vi "Finish.vi"(4 "error in":errorcluster) -> ()   [LabVIEW 2013]
doc: "This VI is called just before exiting. It is expected to close I/O refnum, save collected data, etc."
uses:
  <vilib>/Rock Robotics/WPI/Solenoid/WPI_SolenoidValue.ctl
  <vilib>/Rock Robotics/WPI/RobotDrive/WPI_RobotDriveGetSetRefNum.vi
  <vilib>/Rock Robotics/WPI/Joystick/WPI_JoystickGetSetRefNum.vi
  <vilib>/Rock Robotics/WPI/Solenoid/WPI_SolenoidSetEnum.vi
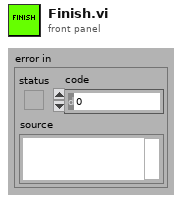
[diagram p1: front panel]
types:
  T1 = typedef "WPI_DigitalInputDevRef.ctl" = cluster{"DevStatus":errorcluster, "DIO Channel":T2, "Digital Module":T3}
  T2 = typedef "FPGA_DIOChannel.ctl" = enum8{"DIO 1", "DIO 2", "DIO 3", "DIO 4", "DIO 5", "DIO 6", "DIO 7", "DIO 8", "DIO 9", "DIO 10", "DIO 11", "DIO 12", "DIO 13", "DIO 14", "Invalid"}
  T3 = typedef "FPGA_TypedefDigitalModule.ctl" = enum16{"Digital Module 1", "Digital Module 2"}
  T4 = typedef "WPI_JoystickDevRef.ctl" = cluster{"Device":T5}
  T5 = typedef "WPI_JoystickDeviceEnum.ctl" = enum16{"USB 1", "USB 2", "USB 3", "USB 4", "Kinect 1", "Kinect 2"}
  T6 = typedef "WPI_CameraDevRef.ctl" = cluster{"Camera Address":string, "CameraStatus":errorcluster, "Acquire Image Notifier":refnum<notifier>}
  T7 = typedef "WPI_RobotDriveDevRef.ctl" = cluster{"DevStatus":errorcluster, "Motors[]":T8[], "Square Inputs":bool, "Max Output":dbl, "Isochronous":bool}
  T8 = typedef "WPI_MotorControlDeviceRef.ctl" = cluster{"DeviceStatus":errorcluster, "Type":enum16{"PWM", "CAN"}, "PWM":cluster{"Digital Module":T3, "PWM Channel":T9, "DeadBand":T10}, "CAN":cluster{"Device Number":u8, "Control Mode":T11, "Semaphore":T12, "Max Vout":dbl}, "Invert":bool, "TransformRef":T13, "InvTransformRef":T13}
  T9 = typedef "FPGA_DIOPWMChannel.ctl" = enum8{"PWM 1", "PWM 2", "PWM 3", "PWM 4", "PWM 5", "PWM 6", "PWM 7", "PWM 8", "PWM 9", "PWM 10", "Invalid"}
  T10 = typedef "WPI_PWMDeadband.ctl" = cluster{"Name":string, "maxPositivePwm":i32, "minPositivePwm":i32, "centerPwm":i32, "maxNegativePwm":i32, "minNegativePwm":i32, "angularRange":u16}
  T11 = typedef "WPI_CANJaguar_ControlMode.ctl" = enum8{"Percent VBus", "Current", "Speed", "Position", "Voltage"}
  T12 = typedef "Semaphore RefNum" = refnum<k1>
  T13 = typedef "WPI_PWMTransform_ConPane.ctl" = refnum<vi>
  T14 = typedef "WPI_EncoderDevRef.ctl" = cluster{"DevStatus":errorcluster, "EncoderIndex":T15, "CounterIndex":T16, "DistancePerCount":dbl, "Decoding Type":T17}
  T15 = typedef "FPGA_EncoderIdx.ctl" = enum8{"Enc 0", "Enc 1", "Enc 2", "Enc 3", "Invalid"}
  T16 = typedef "FPGA_CounterCtrSystemIndex.ctl" = enum8{"Ctr 0", "Ctr 1", "Ctr 2", "Ctr 3", "Ctr 4", "Ctr 5", "Ctr 6", "Ctr 7", "Invalid"}
  T17 = typedef "WPI_EncoderType.ctl" = enum16{"1x", "2x", "4x"}
  T18 = typedef "WPI_SolenoidDevRef.ctl" = cluster{"DevStatus":errorcluster, "Solenoid Module":T19, "Forward Solenoid Channel":T20, "Reverse Solenoid Channel":T20}
  T19 = typedef "FPGA_TypedefSolenoidModule.ctl" = enum16{"Solenoid Module 1", "Solenoid Module 2"}
  T20 = typedef "WPI_SolenoidChannel.ctl" = enum8{"Solenoid 1", "Solenoid 2", "Solenoid 3", "Solenoid 4", "Solenoid 5", "Solenoid 6", "Solenoid 7", "Solenoid 8", "Invalid"}
  T21 = typedef "WPI_SolenoidValue.ctl" = enum16{"Off", "On", "Forward", "Reverse"}
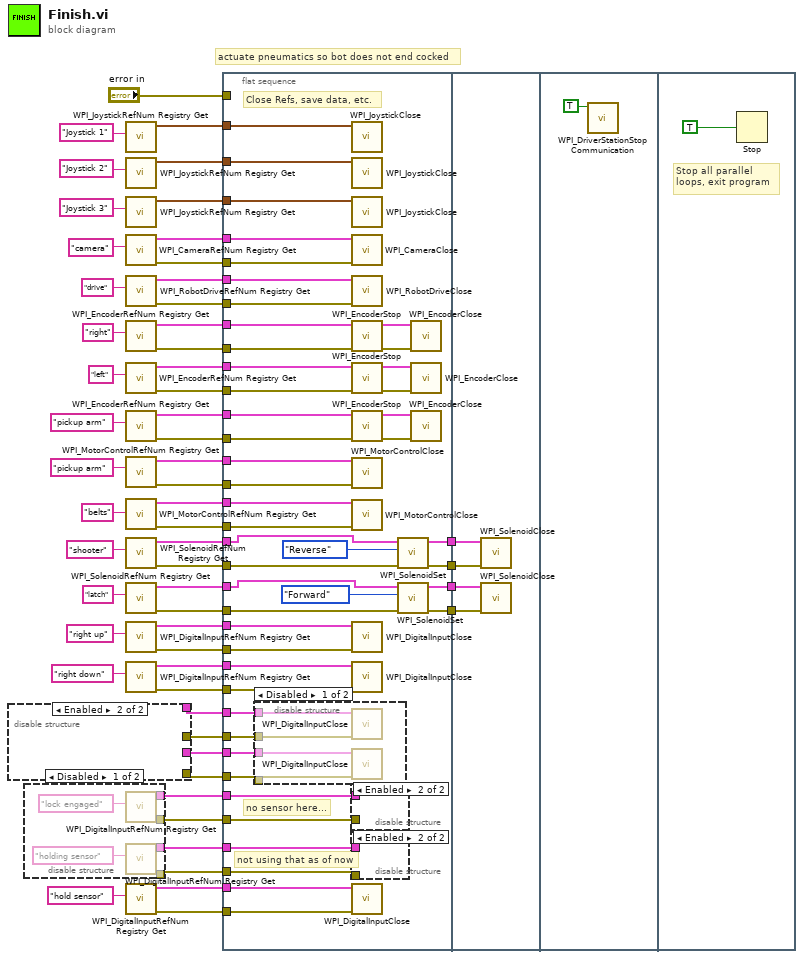
[diagram p0: block diagram]
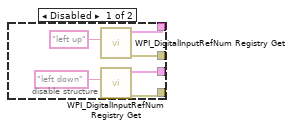
[diagram p2: hidden frame]
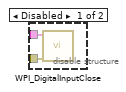
[diagram p5: hidden frame]
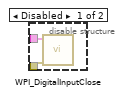
[diagram p6: hidden frame]
diagram:
  # "actuate pneumatics so bot does not end cocked"
  n1 = disable-structure shown="Enabled" {
    disable-tunnel: [w59 _] -> w15
    disable-tunnel: [w58 _] -> w14
    disable-tunnel: [w57 _] -> w13
    disable-tunnel: [w56 _] -> w12
    frame Disabled {
      n2 = call <vilib>:"WPI_DigitalInputRefNum Registry Get.vi"("refnum name"="left up") -> ("error out"=w58:errorcluster, "DigitalInputDevRef"=w59:T1)  [unwired: 9 in]
      n3 = call <vilib>:"WPI_DigitalInputRefNum Registry Get.vi"("refnum name"="left down") -> ("error out"=w56:errorcluster, "DigitalInputDevRef"=w57:T1)  [unwired: 9 in]
    }
    frame Enabled {
    }
  }
  n4 = disable-structure shown="Disabled" {
    disable-tunnel: [w67 _] -> w9
    disable-tunnel: [w66 _] -> w8
    disable-tunnel: [w64 _] -> w6
    disable-tunnel: [w63 _] -> w5
    frame Disabled {
      n5 = call <vilib>:"WPI_DigitalInputRefNum Registry Get.vi"("refnum name"="lock engaged") -> ("error out"=w64:errorcluster, "DigitalInputDevRef"=w63:T1)  [unwired: 9 in]
      n6 = call <vilib>:"WPI_DigitalInputRefNum Registry Get.vi"("refnum name"="holding sensor") -> ("error out"=w67:errorcluster, "DigitalInputDevRef"=w66:T1)  [unwired: 9 in]
    }
    frame Enabled {
    }
  }
  n7 = call <vilib>:"WPI_JoystickRefNum Registry Get.vi"("refnum name"="Joystick 1") -> ("JoystickDevRef"=w54:T4)  [unwired: 1 in, 9 out]
  n8 = call <vilib>:"WPI_JoystickRefNum Registry Get.vi"("refnum name"="Joystick 2") -> ("JoystickDevRef"=w51:T4)  [unwired: 1 in, 9 out]
  n9 = call <vilib>:"WPI_JoystickRefNum Registry Get.vi"("refnum name"="Joystick 3") -> ("JoystickDevRef"=w48:T4)  [unwired: 1 in, 9 out]
  n10 = call <vilib>:"WPI_CameraRefNum Registry Get.vi"("refnum name"="camera") -> ("error out"=w41:errorcluster, "CameraDevRef"=w53:T6)  [unwired: 1 in, 8 out]
  n11 = call <vilib>:"WPI_RobotDriveRefNum Registry Get.vi"("refnum name"="drive") -> ("error out"=w40:errorcluster, "RobotDriveDevRef"=w46:T7)  [unwired: 9 in]
  n12 = call <vilib>:"WPI_EncoderRefNum Registry Get.vi"("refnum name"="right") -> ("error out"=w39:errorcluster, "EncoderDevRef"=w43:T14)  [unwired: 9 in]
  n13 = call <vilib>:"WPI_EncoderRefNum Registry Get.vi"("refnum name"="left") -> ("error out"=w38:errorcluster, "EncoderDevRef"=w42:T14)  [unwired: 9 in]
  n14 = call <vilib>:"WPI_EncoderRefNum Registry Get.vi"("refnum name"="pickup arm") -> ("error out"=w37:errorcluster, "EncoderDevRef"=w35:T14)  [unwired: 9 in]
  n15 = call <vilib>:"WPI_MotorControlRefNum Registry Get.vi"("refnum name"="pickup arm") -> ("error out"=w31:errorcluster, "MotorControlDevRef"=w32:T8)  [unwired: 9 in]
  n16 = call <vilib>:"WPI_MotorControlRefNum Registry Get.vi"("refnum name"="belts") -> ("error out"=w29:errorcluster, "MotorControlDevRef"=w30:T8)  [unwired: 9 in]
  n17 = call <vilib>:"WPI_SolenoidRefNum Registry Get.vi"("refnum name"="shooter") -> ("error out"=w27:errorcluster, "SolenoidDevRef"=w28:T18)  [unwired: 9 in]
  n18 = call <vilib>:"WPI_SolenoidRefNum Registry Get.vi"("refnum name"="latch") -> ("error out"=w23:errorcluster, "SolenoidDevRef"=w24:T18)  [unwired: 9 in]
  n19 = call <vilib>:"WPI_DigitalInputRefNum Registry Get.vi"("refnum name"="right up") -> ("error out"=w18:errorcluster, "DigitalInputDevRef"=w19:T1)  [unwired: 9 in]
  n20 = call <vilib>:"WPI_DigitalInputRefNum Registry Get.vi"("refnum name"="right down") -> ("error out"=w16:errorcluster, "DigitalInputDevRef"=w17:T1)  [unwired: 9 in]
  n21 = call <vilib>:"WPI_DigitalInputRefNum Registry Get.vi"("refnum name"="hold sensor") -> ("error out"=w11:errorcluster, "DigitalInputDevRef"=w10:T1)  [unwired: 9 in]
  n22 = flat-sequence {
    tunnel: w54 -> [w114]
    tunnel: w53 -> [w113]
    tunnel: w51 -> [w112]
    tunnel: w48 -> [w111]
    tunnel: w46 -> [w110]
    tunnel: w43 -> [w109]
    tunnel: w42 -> [w102]
    tunnel: w41 -> [w106]
    tunnel: w40 -> [w105]
    tunnel: w39 -> [w104]
    tunnel: w38 -> [w103]
    tunnel: w37 -> [w98]
    tunnel: w35 -> [w97]
    tunnel: w32 -> [w95]
    tunnel: w31 -> [w94]
    tunnel: w30 -> [w92]
    tunnel: w29 -> [w93]
    tunnel: w28 -> [w72]
    tunnel: w27 -> [w74]
    tunnel: w24 -> [w76]
    tunnel: w23 -> [w75]
    tunnel: "error in" -> [_]
    tunnel: w19 -> [w87]
    tunnel: w18 -> [w88]
    tunnel: w17 -> [w86]
    tunnel: w16 -> [w89]
    tunnel: w15 -> [w85]
    tunnel: w14 -> [w90]
    tunnel: w13 -> [w84]
    tunnel: w12 -> [w91]
    tunnel: w8 -> [w82]
    tunnel: w9 -> [w81]
    tunnel: w10 -> [w83]
    tunnel: w11 -> [w80]
    tunnel: w5 -> [w79]
    tunnel: w6 -> [w78]
    tunnel: [w71] -> w4
    tunnel: [w70] -> w3
    tunnel: [w69] -> w2
    tunnel: [w68] -> w1
    tunnel: w4 -> [w124]
    tunnel: w3 -> [w123]
    tunnel: w2 -> [w125]
    tunnel: w1 -> [w126]
    frame #0 {
      # "no sensor here..."
      # "not using that as of now"
      # "Close Refs, save data, etc."
      n23 = disable-structure shown="Disabled" {
        disable-tunnel: w91 -> [w118 _]
        disable-tunnel: w90 -> [w117 _]
        disable-tunnel: w85 -> [w116 _]
        disable-tunnel: w84 -> [w115 _]
        frame Disabled {
          n24 = call <vilib>:"WPI_DigitalInputClose.vi"("error in (no error)"=w117, "DigitalInputDevRef"=w116) -> ()  [unwired: 9 in, 1 out]
          n25 = call <vilib>:"WPI_DigitalInputClose.vi"("error in (no error)"=w118, "DigitalInputDevRef"=w115) -> ()  [unwired: 9 in, 1 out]
        }
        frame Enabled {
        }
      }
      n26 = call <vilib>:"WPI_JoystickClose.vi"("JoystickDevRef"=w114) -> ()  [unwired: 11 out]
      n27 = call <vilib>:"WPI_JoystickClose.vi"("JoystickDevRef"=w112) -> ()  [unwired: 11 out]
      n28 = call <vilib>:"WPI_JoystickClose.vi"("JoystickDevRef"=w111) -> ()  [unwired: 11 out]
      n29 = call <vilib>:"WPI_CameraClose.vi"("error in (no error)"=w106, "CameraDevRef"=w113) -> ()  [unwired: 10 out]
      n30 = call <vilib>:"WPI_RobotDriveClose.vi"("error in (no error)"=w105, "RobotDriveDevRef"=w110) -> ()  [unwired: 9 in, 1 out]
      n31 = call <vilib>:"WPI_EncoderStop.vi"("error in (no error)"=w104, "EncoderDevRef"=w109) -> ("error out"=w108:errorcluster, "EncoderDevRef"=w107:T14)  [unwired: 8 in]
      n32 = call <vilib>:"WPI_EncoderStop.vi"("error in (no error)"=w103, "EncoderDevRef"=w102) -> ("error out"=w100:errorcluster, "EncoderDevRef"=w101:T14)  [unwired: 8 in]
      n33 = call <vilib>:"WPI_EncoderStop.vi"("error in (no error)"=w98, "EncoderDevRef"=w97) -> ("error out"=w99:errorcluster, "EncoderDevRef"=w96:T14)  [unwired: 8 in]
      n34 = call <vilib>:"WPI_MotorControlClose.vi"("error in (no error)"=w94, "MotorControlDevRef"=w95) -> ()  [unwired: 9 in, 1 out]
      n35 = call <vilib>:"WPI_MotorControlClose.vi"("error in (no error)"=w93, "MotorControlDevRef"=w92) -> ()  [unwired: 9 in, 1 out]
      n36 = call <vilib>:"WPI_DigitalInputClose.vi"("error in (no error)"=w88, "DigitalInputDevRef"=w87) -> ()  [unwired: 9 in, 1 out]
      n37 = call <vilib>:"WPI_DigitalInputClose.vi"("error in (no error)"=w89, "DigitalInputDevRef"=w86) -> ()  [unwired: 9 in, 1 out]
      n38 = disable-structure shown="Enabled" {
        disable-tunnel: w79 -> [w120 _]
        disable-tunnel: w78 -> [w119 _]
        frame Disabled {
          n39 = call <vilib>:"WPI_DigitalInputClose.vi"("error in (no error)"=w119, "DigitalInputDevRef"=w120) -> ()  [unwired: 9 in, 1 out]
        }
        frame Enabled {
        }
      }
      n40 = disable-structure shown="Enabled" {
        disable-tunnel: w82 -> [w122 _]
        disable-tunnel: w81 -> [w121 _]
        frame Disabled {
          n41 = call <vilib>:"WPI_DigitalInputClose.vi"("error in (no error)"=w121, "DigitalInputDevRef"=w122) -> ()  [unwired: 9 in, 1 out]
        }
        frame Enabled {
        }
      }
      n42 = call <vilib>:"WPI_DigitalInputClose.vi"("error in (no error)"=w80, "DigitalInputDevRef"=w83) -> ()  [unwired: 9 in, 1 out]
      n43 = call-poly <vilib>:"WPI_SolenoidSet.vi"("error in (no error)"=w74, "Value"=WPI_SolenoidValue."Reverse", "SolenoidDevRef"=w72) -> ("error out"=w69:errorcluster, "SolenoidDevRef"=w68:T18)  [unwired: 7 in]
      n44 = call-poly <vilib>:"WPI_SolenoidSet.vi"("error in (no error)"=w75, "Value"=WPI_SolenoidValue."Forward", "SolenoidDevRef"=w76) -> ("error out"=w70:errorcluster, "SolenoidDevRef"=w71:T18)  [unwired: 7 in]
      n45 = call <vilib>:"WPI_EncoderClose.vi"("error in (no error)"=w108, "EncoderDevRef"=w107) -> ()  [unwired: 9 in, 1 out]
      n46 = call <vilib>:"WPI_EncoderClose.vi"("error in (no error)"=w100, "EncoderDevRef"=w101) -> ()  [unwired: 9 in, 1 out]
      n47 = call <vilib>:"WPI_EncoderClose.vi"("error in (no error)"=w99, "EncoderDevRef"=w96) -> ()  [unwired: 9 in, 1 out]
    }
    frame #1 {
      n48 = call <vilib>:"WPI_SolenoidClose.vi"("error in (no error)"=w125, "SolenoidDevRef"=w126) -> ()  [unwired: 9 in, 1 out]
      n49 = call <vilib>:"WPI_SolenoidClose.vi"("error in (no error)"=w123, "SolenoidDevRef"=w124) -> ()  [unwired: 9 in, 1 out]
    }
    frame #2 {
      n50 = call <vilib>:"WPI_DriverStationStop Communication.vi"("StopCommunication"=TRUE) -> ()  [unwired: 10 in, 1 out]
    }
    frame #3 {
      # "Stop all parallel\nloops, exit program"
      n51 = Stop(stop? (T)=TRUE ("Quit")) -> ()
    }
  }
